vi "GetSettingsFileFromTargetSetNum.vi"(5 "target set #":i32, 6 "# Cycles":i16=20, 7 "Block":T1(array[cluster])) -> (0 "# target sets":u16, 1 "Completed list?":bool, 2 "apply new settings?":bool, 3 "Settings file":path)   [LabVIEW 2010]
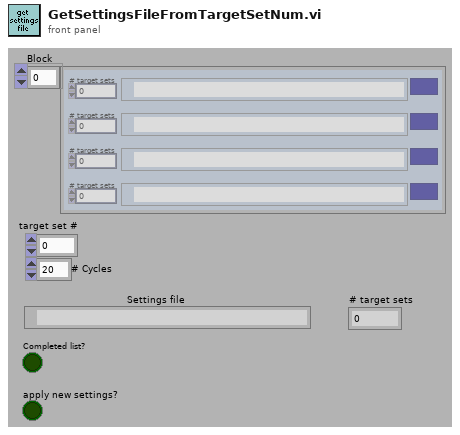
[diagram p1: front panel]
types:
  T1 = cluster{"Settings file":path, "# target sets":u16}[]
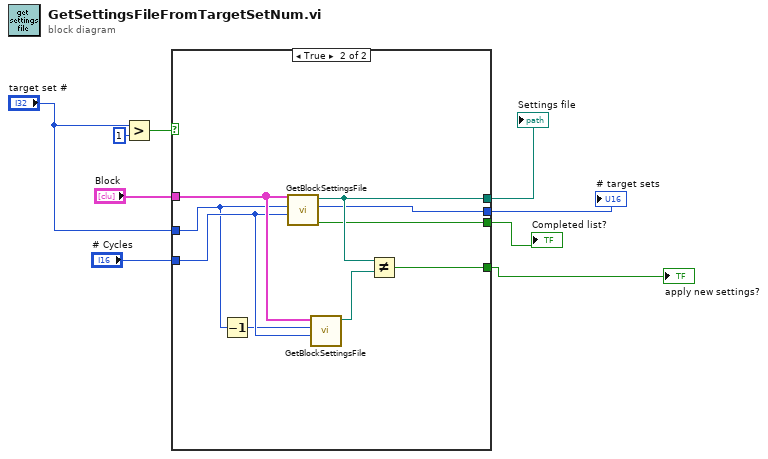
[diagram p0: block diagram]
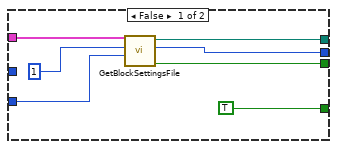
[diagram p2: hidden frame]
diagram:
  n1 = Greater?(x="target set #", y=1) -> (0:w9:bool)
  n2 = case shown="True" w9 {
    tunnel: "Block" -> [w16 w25]
    tunnel: "# Cycles" -> [w15 w24]
    tunnel: [w13 w21] -> w6
    tunnel: [w12 w18] -> w3
    tunnel: "target set #" -> [_ w23]
    tunnel: [TRUE w17] -> w1
    tunnel: [w10 w19] -> w4
    frame False {
      n3 = call "GetBlockSettingsFile.vi"("# Cycles"=w15, "target set #"=1 ("y"), "Block"=w16) -> ("Completed list?"=w12:bool, "# target sets"=w10:i16, "Settings file"=w13:path)  [unwired: 2 in]
    }
    frame True {
      n4 = Decrement(x=w23) -> (x-1=w22:i32)
      n5 = call "GetBlockSettingsFile.vi"("# Cycles"=w24, "target set #"=w23, "Block"=w25) -> ("Completed list?"=w18:bool, "# target sets"=w19:i16, "Settings file"=w21:path)  [unwired: 2 in]
      n6 = call "GetBlockSettingsFile.vi"("# Cycles"=w24, "target set #"=w22, "Block"=w25) -> ("Settings file"=w20:path)  [unwired: 2 in, 2 out]
      n7 = Not Equal?(x=w21, y=w20) -> (x != y?=w17:bool)
    }
  }
  "Settings file" <- w6
  "Completed list?" <- w3
  "# target sets" <- w4
  "apply new settings?" <- w1
